vi "Pockels Cal-Exctract cal subset indexes.vi"(11 "Pockels Cal table":string[][](array[string])) -> (3 "Cal subset indexes":T1)   [LabVIEW 2020]
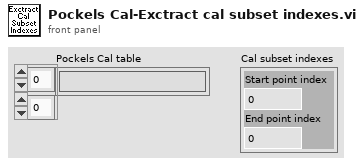
[diagram p1: front panel]
types:
  T1 = cluster{"Start point index":i32, "End point index":i32}
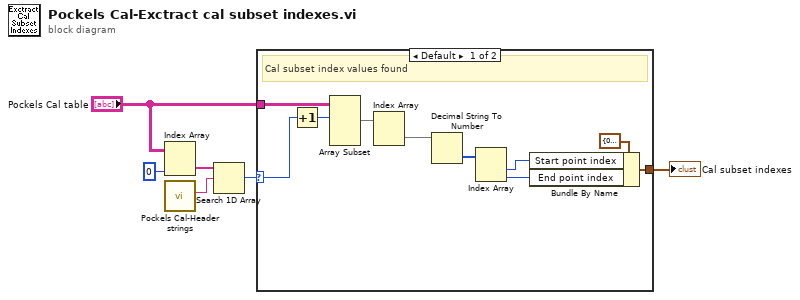
[diagram p0: block diagram]
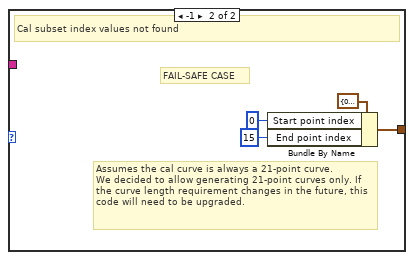
[diagram p2: hidden frame]
diagram:
  n1 = Index Array(array="Pockels Cal table", index (col)=0 ("disabled index (col)")) -> (element=w5:string[])  [unwired: 1 in]
  n2 = call "Pockels Cal-Header strings.vi"() -> ("Cal subset indexes header string"=w6:string)  [unwired: 9 in, 2 out]
  n3 = Search 1D Array(1D array=w5, element=w6) -> (index of element=w2:i32)  [unwired: 1 in]
  n4 = case shown="Default" w2 {
    selector: w2 -> [w16 _]
    tunnel: "Pockels Cal table" -> [w7 _]
    tunnel: [w8 w19] -> w1
    frame Default {
      # "Cal subset index values found"
      n5 = Increment(x=w16) -> (x+1=w15:i32)
      n6 = Array Subset(array=w7, index (row)=w15) -> (w14:string[][])  [unwired: 3 in]
      n7 = Index Array(array=w14) -> (element=w13:string[])  [unwired: 2 in]
      n8 = Decimal String To Number(string=w13) -> (number=w11:i32[])  [unwired: 2 in, 1 out]
      n9 = Index Array(array=w11) -> (element #1=w10:i32, element #2=w9:i32)  [unwired: 2 in]
      n10 = Bundle By Name(cluster=T1 {"Start point index"=0, "End point index"=11} ("Cal subset indexes"), "Start point index"=w10, "End point index"=w9) -> (w8:T1)
    }
    frame -1 {
      # "FAIL-SAFE CASE"
      # "Assumes the cal curve is always a 21-point curve.\nWe decided to allow generating 21-point curves only. If the curve length requirement changes in the future, this code will need to be upgraded."
      # "Cal subset index values not found"
      n11 = Bundle By Name(cluster=T1 {"Start point index"=0, "End point index"=11} ("Cal subset indexes"), "Start point index"=0, "End point index"=15) -> (w19:T1)
    }
  }
  "Cal subset indexes" <- w1
